vi "Bilaterate.vi"() -> ()   [LabVIEW 2015]
panel:
  out "Y":dbl
  out "X":dbl
  in  "B":cluster{"X":dbl, "Y":dbl, "Dist":dbl}
  in  "A":cluster{"X":dbl, "Y":dbl, "Dist":dbl}
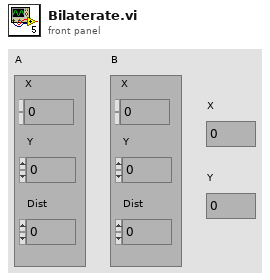
[diagram p1: front panel]
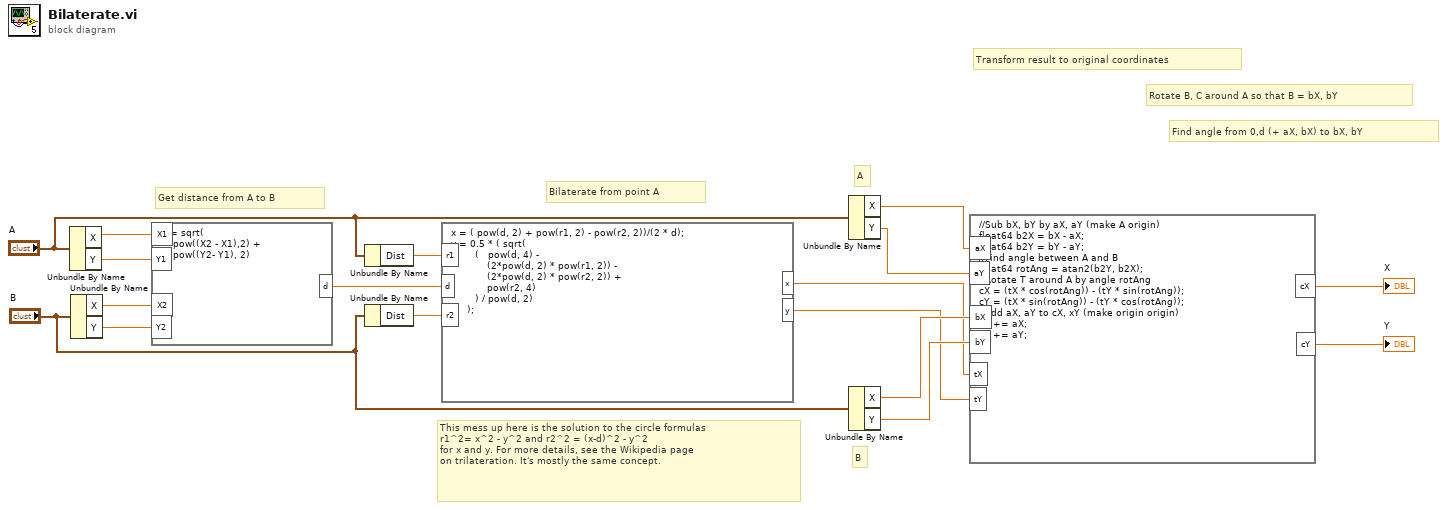
[diagram p0: block diagram]
diagram:
  # "Find angle from 0,d (+ aX, bX) to bX, bY"
  # "B"
  # "A"
  # "Rotate B, C around A so that B = bX, bY"
  # "This mess up here is the solution to the circle formulas\nr1^2= x^2 - y^2 and r2^2 = (x-d)^2 - y^2\nfor x and y. For more details, see the Wikipedia page\non trilateration. It's mostly the same concept."
  # "Transform result to original coordinates"
  # "Bilaterate from point A"
  # "Get distance from A to B"
  n1 = Unbundle By Name("A") -> ("X"=w17:dbl, "Y"=w16:dbl)
  n2 = Unbundle By Name("B") -> ("X"=w15:dbl, "Y"=w14:dbl)
  n3 = formula code="d = sqrt(\n    pow((X2 - X1),2) +\n    pow((Y2- Y1), 2)\n);"("X1"=w17, "Y1"=w16, "X2"=w15, "Y2"=w14) -> ("d"=w9:dbl)
  n4 = Unbundle By Name("A") -> ("Dist"=w12:dbl)
  n5 = Unbundle By Name("B") -> ("Dist"=w13:dbl)
  n6 = formula code="x = ( pow(d, 2) + pow(r1, 2) - pow(r2, 2))/(2 * d);\ny = 0.5 * ( sqrt(\n        (   pow(d, 4) -\n            (2*pow(d, 2) * pow(r1, 2)) -\n            (2*pow(d, 2) * pow(r2, 2)) +\n            pow(r2, 4)\n        ) / pow(d, 2)\n)    );"("r1"=w12, "r2"=w13, "d"=w9) -> ("x"=w2:dbl, "y"=w1:dbl)
  n7 = Unbundle By Name("A") -> ("X"=w6:dbl, "Y"=w5:dbl)
  n8 = Unbundle By Name("B") -> ("X"=w4:dbl, "Y"=w3:dbl)
  n9 = formula code="//Sub bX, bY by aX, aY (make A origin)\nfloat64 b2X = bX - aX;\nfloat64 b2Y = bY - aY;\n//Find angle between A and B\nfloat64 rotAng = atan2(b2Y, b2X);\n//Rotate T around A by angle rotAng\ncX = (tX * cos(rotAng)) - (tY * sin(rotAng)); \ncY = (tX * sin(rotAng)) - (tY * cos(rotAng));\n//Add aX, aY to cX, xY (make origin origin)\ncX += aX;\ncY += aY;"("aX"=w6, "aY"=w5, "bX"=w4, "bY"=w3, "tX"=w2, "tY"=w1) -> ("cX"=→"X":dbl, "cY"=→"Y":dbl)
